vi "test_Checksum U8 - Check Protection.vi"(8 "error in (no error)":errorcluster) -> (0 "error out":errorcluster)   [LabVIEW 2019, in "Protections Unit Tests.lvclass"]
uses:
  Protections Unit Tests.lvclass
  Checksum U8/Checksum U8.lvclass
  <vilib>/addons/_JKI Toolkits/VI Tester/TestCase.llb/TestCase.lvclass
  C:/Program Files (x86)/National Instruments/LabVIEW 2019/vi.lib/addons/_JKI Toolkits/VI Tester/TestCase.llb/TestCase.lvclass
panel:
  out "Checksum U8 out":refnum<class "Checksum U8.lvclass">
  in  "Checksum U8 in":refnum<class "Checksum U8.lvclass">
  out "TestCase out":refnum<class "Protections Unit Tests.lvclass">
  in  "TestCase in":refnum<class "Protections Unit Tests.lvclass">
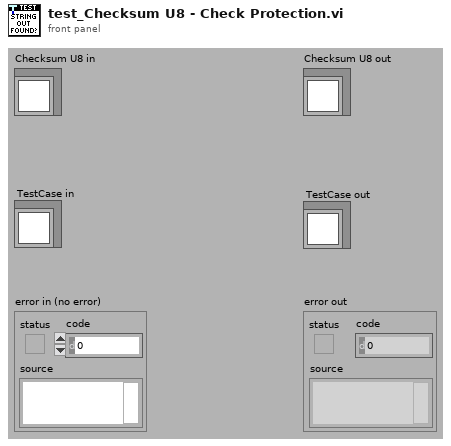
[diagram p1: front panel]
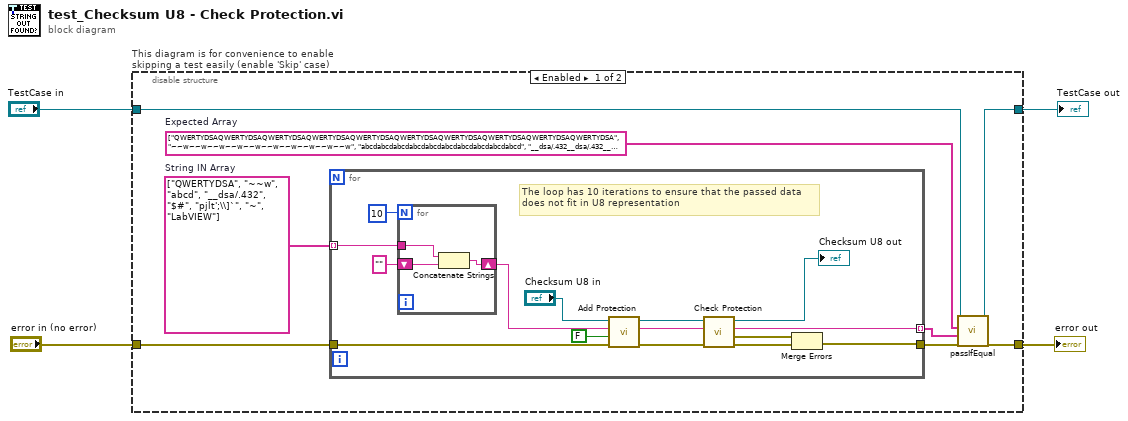
[diagram p0: block diagram]
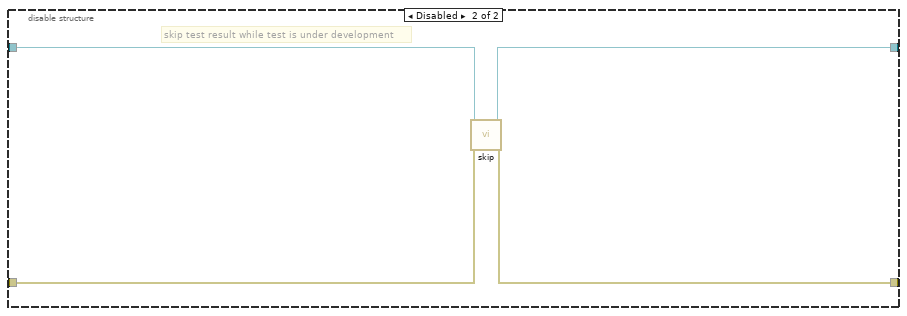
[diagram p2: hidden frame]
diagram:
  n1 = disable-structure "This diagram is for convenience to enable skipping a test easily (enable 'Skip' case)" shown="Enabled" {
    disable-tunnel: "TestCase in" -> [w10 w34]
    disable-tunnel: [w11 w32] -> w1
    disable-tunnel: [w12 w33] -> w3
    disable-tunnel: "error in (no error)" -> [w9 w31]
    frame Enabled {
      w5 = string[] ["QWERTYDSAQWERTYDSAQWERTYDSAQWERTYDSAQWERTYDSAQWERTYDSAQWERTYDSAQWERTYDSAQWERTYDSAQWERTYDSA", "~~w~~w~~w~~w~~w~~w~~w~~w~~w~~w", "abcdabcdabcdabcdabcdabcdabcdabcdabcdabcd", "__dsa/.432__dsa/.432__dsa/.432__dsa/.432__dsa/.432__dsa/.432__dsa/.432__dsa/.432__dsa/.432__dsa/.432", "$#$#$#$#$#$#$#$#$#$#", "pjlt';\\]`pjlt';\\]`pjlt';\\]`pjlt';\\]`pjlt';\\]`pjlt';\\]`pjlt';\\]`pjlt';\\]`pjlt';\\]`pjlt';\\]`", "~~~~~~~~~~", "LabVIEWLabVIEWLabVIEWLabVIEWLabVIEWLabVIEWLabVIEWLabVIEWLabVIEWLabVIEW"]  # Expected Array
      w6 = string[] ["QWERTYDSA", "~~w", "abcd", "__dsa/.432", "$#", "pjlt';\\]`", "~", "LabVIEW"]  # String IN Array
      n2 = for {
        tunnel: w6 -> [w25] mode=indexing
        tunnel: w9 -> [w24]
        tunnel: [w14] -> w7
        tunnel: [w17] -> w8 mode=indexing
        # "The loop has 10 iterations to ensure that the passed data\ndoes not fit in U8 representation"
        n3 = for {
          N: 10 -> [_]
          shift-right: [w30] -> w23
          shift-left: "" -> [w29]
          tunnel: w25 -> [w28]
          n4 = Concatenate Strings(w28, w29) -> (w30:string)
        }
        n5 = call-dynamic "Add Protection.vi"("error in (no error)"=w24, "Pad"=FALSE, "String in"=w23, "Checksum U8 in"="Checksum U8 in") -> ("error out"=w18:errorcluster, "String out"=w19:string, "Checksum U8 out"=w21:refnum<class "Checksum U8.lvclass">)  [unwired: 5 in]
        n6 = call-dynamic "Check Protection.vi"("error in (no error)"=w18, "String in"=w19, "Checksum U8 in"=w21) -> ("error out"=w15:errorcluster, "Protection Error"=w16:errorcluster, "String out"=w17:string, "Checksum U8 out"=→"Checksum U8 out":refnum<class "Checksum U8.lvclass">)  [unwired: 5 in]
        n7 = Merge Errors(w16, w15) -> (w14:errorcluster)
      }
      n8 = call-dynamic "passIfEqual.vi"("error in (no error)"=w7, "y"=w8, "x"=w5, "TestCase in"=w10) -> ("error out"=w12:errorcluster, "TestCase out"=w11:refnum<class "Protections Unit Tests.lvclass">)  [unwired: 6 in]
    }
    frame Disabled {
      # "skip test result while test is under development"
      n9 = call <vilib>:"skip.vi"("error in (no error)"=w31, "TestCase in"=w34) -> ("error out"=w33:errorcluster, "TestCase out"=w32:refnum<class "Protections Unit Tests.lvclass">)  [unwired: 8 in]
    }
  }
  "error out" <- w3
  "TestCase out" <- w1
